vi "Process Falling Edge Trigger.vi"(10 "Log File Index":i32, 11 "File Logging Specs in":T1[](array[typedef]) {"File Node Ref" format="%.0x"}) -> (3 "File Logging Specs out":T1[](array[typedef]) {"File Node Ref" format="%.0x"})   [LabVIEW 2027, in "Embedded Data Logger Engine.lvlib"]
uses:
  Embedded Data Logger Engine.lvlib
  File Logging Specification.ctl
  Group Logging Specification.ctl
  Group Buffer Data.ctl
  Property Specification.ctl
  <vilib>/NI VeriStand/Custom Device API/Custom Device Item Ref.ctl
  Shared/Segment Files By.ctl
  Logging State.ctl
  <vilib>/NI VeriStand/Custom Device API/Custom Device API.lvlib
  Shared/Embedded Data Logger Shared.lvlib
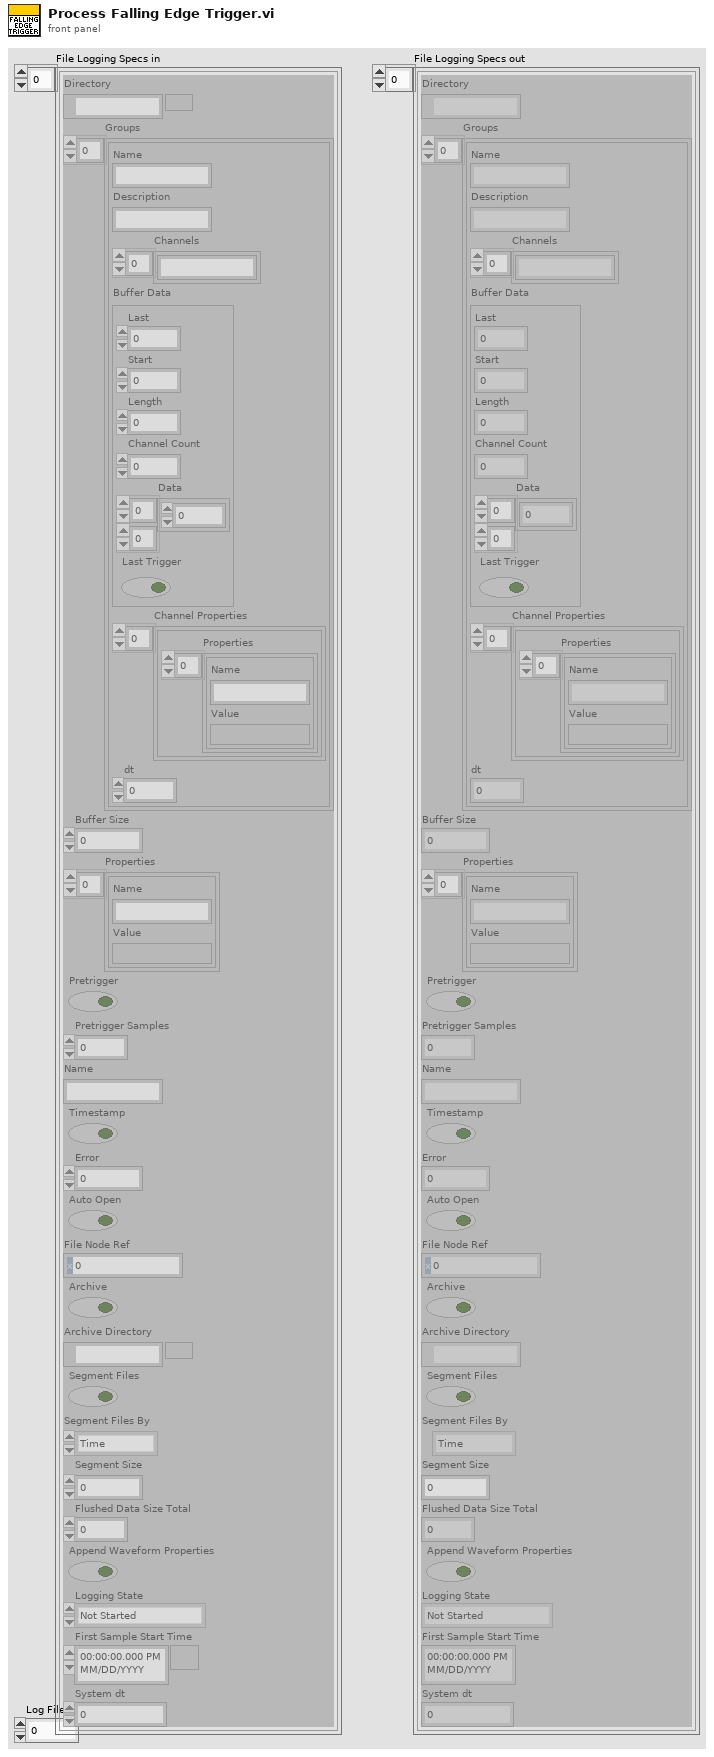
[diagram p1: front panel]
types:
  T1 = typedef "Embedded Data Logger Engine.lvlib/File Logging Specification.ctl" = cluster{"Directory":path, "Groups":T2[], "Buffer Size":i32, "Properties":T4[], "Pretrigger":bool, "Pretrigger Samples":i32, "Name":string, "Timestamp":bool, "Error":i32, "Auto Open":bool, "File Node Ref":T5, "Archive":bool, "Archive Directory":path, "Segment Files":bool, "Segment Files By":T6, "Segment Size":u32, "Flushed Data Size Total":u32, "Append Waveform Properties":bool, "Logging State":T7, "First Sample Start Time":timestamp, "System dt":dbl}
  T2 = typedef "Embedded Data Logger Engine.lvlib/Group Logging Specification.ctl" = cluster{"Name":string, "Description":string, "Channels":string[], "Buffer Data":T3, "Channel Properties":cluster{"Properties":T4[]}[], "dt":dbl}
  T3 = typedef "Embedded Data Logger Engine.lvlib/Group Buffer Data.ctl" = cluster{"Last":i32, "Start":i32, "Length":i32, "Channel Count":i32, "Data":dbl[][], "Last Trigger":bool}
  T4 = typedef "Embedded Data Logger Engine.lvlib/Property Specification.ctl" = cluster{"Name":string, "Value":variant}
  T5 = typedef "Custom Device API.lvlib/Custom Device Item Ref.ctl" = u64
  T6 = typedef "Embedded Data Logger Shared.lvlib/Segment Files By.ctl" = enum16{"Time", "Size"}
  T7 = typedef "Embedded Data Logger Engine.lvlib/Logging State.ctl" = enum16{"Not Started", "Continous Logging", "Paused", "Discontinous Logging"}
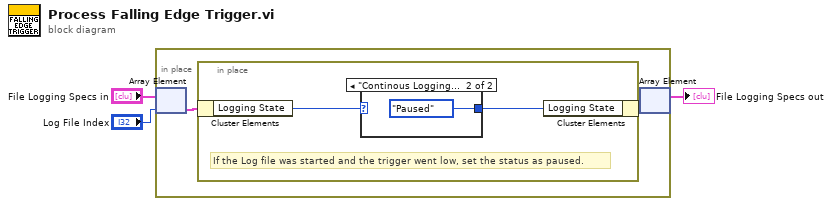
[diagram p0: block diagram]
diagram:
  n1 = in-place {
    n2 = in-place-array #1("File Logging Specs in", "Log File Index") -> (w5:T1)
    n3 = in-place {
      # "If the Log file was started and the trigger went low, set the status as paused."
      n4 = in-place-cluster #2(w5) -> ("Logging State"=w7:T7)
      n5 = case shown="\"Continous Logging\"" w7 {
        selector: w7 -> [w8 _]
        tunnel: [w8 Logging_State."Paused" ("Logging State")] -> w6
        frame Default {
        }
        frame "Continous Logging" {
        }
      }
      n6 = in-place-cluster #2("Logging State"=w6) -> (w4:T1)
    }
    n7 = in-place-array #1(w4) -> (→"File Logging Specs out":T1[])  [unwired: 1 out]
  }
